vi "MB set ID.vi"() -> ()   [LabVIEW 2019]
panel:
  in  "Set":bool
  in  "Cancel Button":bool
  in  "Set and exit":bool
  out "error out":errorcluster
  in  "Select the serial port":refnum<visa-resource-name>
  in  "Unit ID":u8=1 min=1 max=247 step=1
  # "To set the unit ID on a modbus device\n1) Turn off or disconnect all other devices so that ProCoDA is only communicating with ONE DEVICE! This is important because the command to change the address is broadcast to all devices on the Modbus network.\n2) Select the serial port that is connected to the Modbus network\n3) Select the Unit ID that you would like for the one device that is connected to the Modbus network\n4 Hit Okay!\n5) Confirm that the device has accepted the unit ID. Golander 50S pumps  display the unit ID on startup."
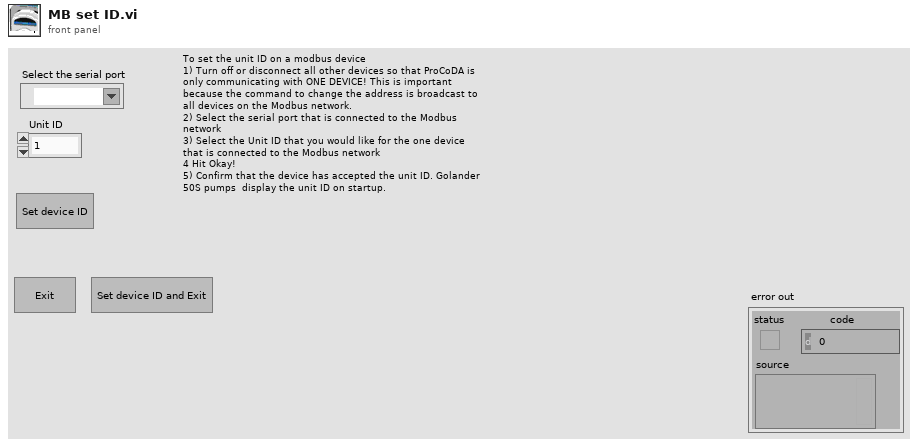
[diagram p1: front panel]
types:
  T1 = cluster{"Mode":enum16{"RTU", "ASCII"}, "Slave Address":u8}
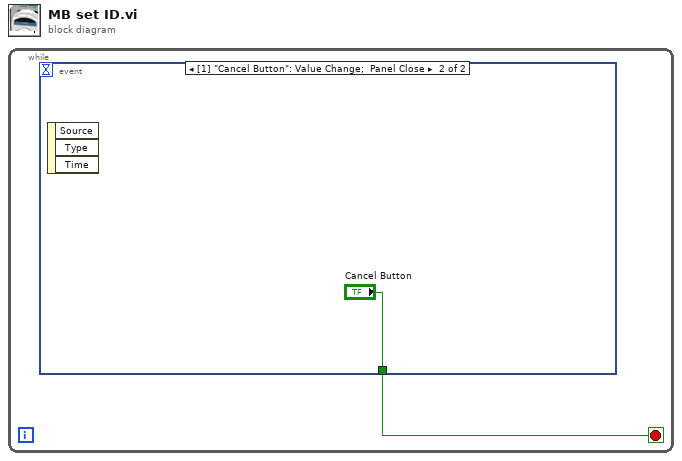
[diagram p0: block diagram]
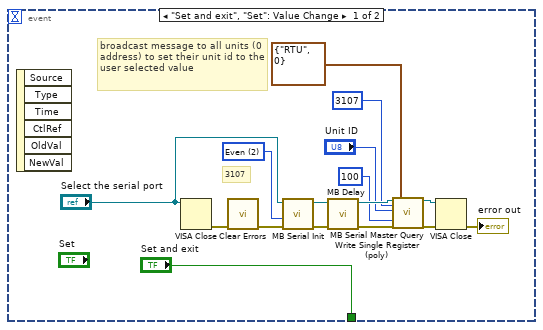
[diagram p2: hidden frame]
diagram:
  n1 = while {
    stop <- w1 stop-if-true
    n2 = event shown="[1] \"Cancel Button\": Value Change;  Panel Close" {
      selector: _ -> [_ _]
      dyn-events: _ -> [_ _]
      timeout: _ -> [_ _]
      tunnel: ["Set and exit" "Cancel Button"] -> w1
      event "Set and exit", "Set": Value Change {
        w17 = u16 2 items=["None", "Odd", "Even", "Mark", "Space"] ("Parity")
        # "broadcast message to all units (0 address) to set their unit id to the user selected value"
        # "3107"
        n3 = event-data() -> ()  [unwired: 1 in, 6 out]
        n4 = VISA Close(VISA resource name="Select the serial port") -> (error out=w7:errorcluster)  [unwired: 1 in]
        n5 = call <vilib>:"Clear Errors.vi"("error in (no error)"=w7) -> ("error out"=w6:errorcluster)  [unwired: 5 in, 1 out]
        n6 = call "MB Serial Init.vi"("error in (no error)"=w6, "Parity"=w17, "VISA resource name"="Select the serial port") -> ("error out"=w15:errorcluster, "VISA resource name out"=w16:refnum<visa-resource-name>)  [unwired: 7 in]
        n7 = call "MB Delay.vi"("error in (no error)"=w15, "VISA Refnum in"=w16) -> ("error out"=w13:errorcluster, "VISA Refnum out"=w14:refnum<visa-resource-name>)  [unwired: 8 in]
        n8 = call "MB Serial Master Query Write Single Register (poly).vi"("VISA resource name"=w14, "Address"=u16 3107, "Holding Register"="Unit ID", "Timeout"=u32 100, "error in"=w13, "Serial Parameters"=T1 {"Mode"=enum."RTU", "Slave Address"=0}) -> ("VISA resource name out"=w4:refnum<visa-resource-name>, "error out"=w3:errorcluster)  [unwired: 11 in, 1 out]
        n9 = VISA Close(VISA resource name=w4, error in (no error)=w3) -> (error out=→"error out":errorcluster)
      }
      event "Cancel Button": Value Change; Panel Close {
        n10 = event-data() -> ()  [unwired: 1 in, 3 out]
      }
    }
  }
